vi "APS line v.vi"(0 "Dimension":i32, 1 "TransPara":dbl, 2 "Wait":cluster{"h_event":u32, "i32_ret":i32}, 5 "Axis_ID_Array":i32, 7 "Option":i32, 9 "PositionArray":dbl, 11 "error in (no error)":errorcluster caption="错误输入（无错误）", 12 "Vm":dbl) -> (3 "TransPara out":dbl, 4 "Wait out":cluster{"h_event":u32, "i32_ret":i32}, 6 "Axis_ID_Array out":i32, 8 "function return":i32, 10 "PositionArray out":dbl, 15 "error out":errorcluster caption="错误输出")   [LabVIEW 2011, in "APS168.lvlib"]
doc: "I32 FNTYPE APS_line_v( I32 Dimension, I32 *Axis_ID_Array, I32 Option, F64 *PositionArray, F64 *TransPara, F64 Vm, ASYNCALL *Wait);"
uses:
  APS168.lvlib
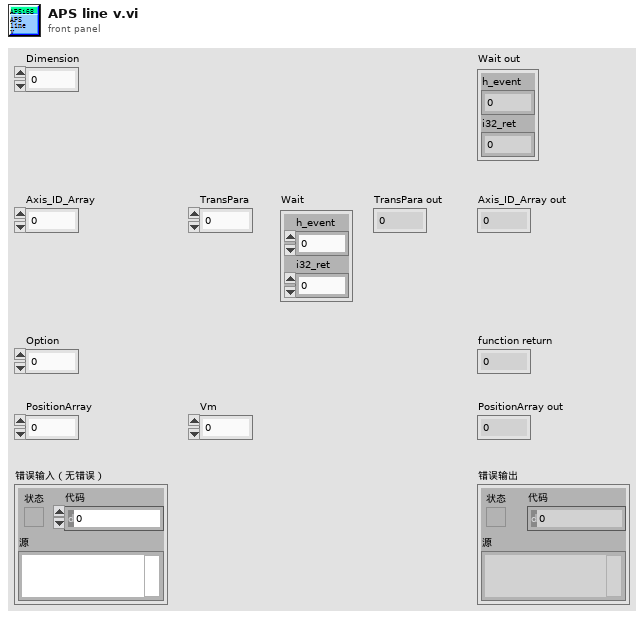
[diagram p1: front panel]
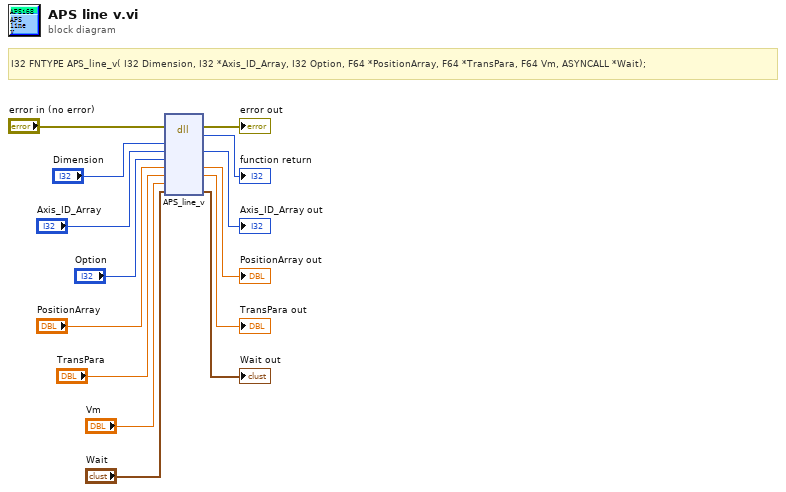
[diagram p0: block diagram]
diagram:
  # "I32 FNTYPE APS_line_v( I32 Dimension, I32 *Axis_ID_Array, I32 Option, F64 *PositionArray, F64 *TransPara, F64 Vm, ASYNCALL *Wait);"
  n1 = dll-call lib="PTH1Labs E软件ADLINK 204CAPS_1_7_1_LIB line 连续运动204APS168.*" fn="APS_line_v"(error in="error in (no error)", "Dimension"="Dimension", "Axis_ID_Array"="Axis_ID_Array", "Option"="Option", "PositionArray"="PositionArray", "TransPara"="TransPara", "Vm"="Vm", "Wait"="Wait") -> (error out=→"error out":errorcluster, →"function return":i32, "Axis_ID_Array"=→"Axis_ID_Array out":i32, "PositionArray"=→"PositionArray out":dbl, "TransPara"=→"TransPara out":dbl, "Wait"=→"Wait out":cluster{"h_event":u32, "i32_ret":i32})  [unwired: 5 in, 1 out]
